vi "Untitled 8.vi"() -> ()   [LabVIEW 2009]
uses:
  <vilib>/Utility/file.llb/Read From Spreadsheet File (DBL).vi
  <vilib>/Analysis/NI_AALBase.lvlib
panel:
  in  "butter?":bool
  in  "w":dbl
  out "x/y 2":dbl
  out "x/y":dbl
  out "output cluster 3":cluster{"locations":dbl[], "locations":dbl[]}(graph)
  out "output cluster 2":cluster{"locations":dbl[], "amplitudes":dbl[]}[](graph)
  in  "threshold":dbl
  in  "offset":dbl
  in  "method":i32(ring)=1 items=["median", "noise center", "Minimum"]
  in  "number of rows (all:-1)":i32=300
  out "all rows":dbl[][](graph)
  in  "file path (dialog if empty)":path
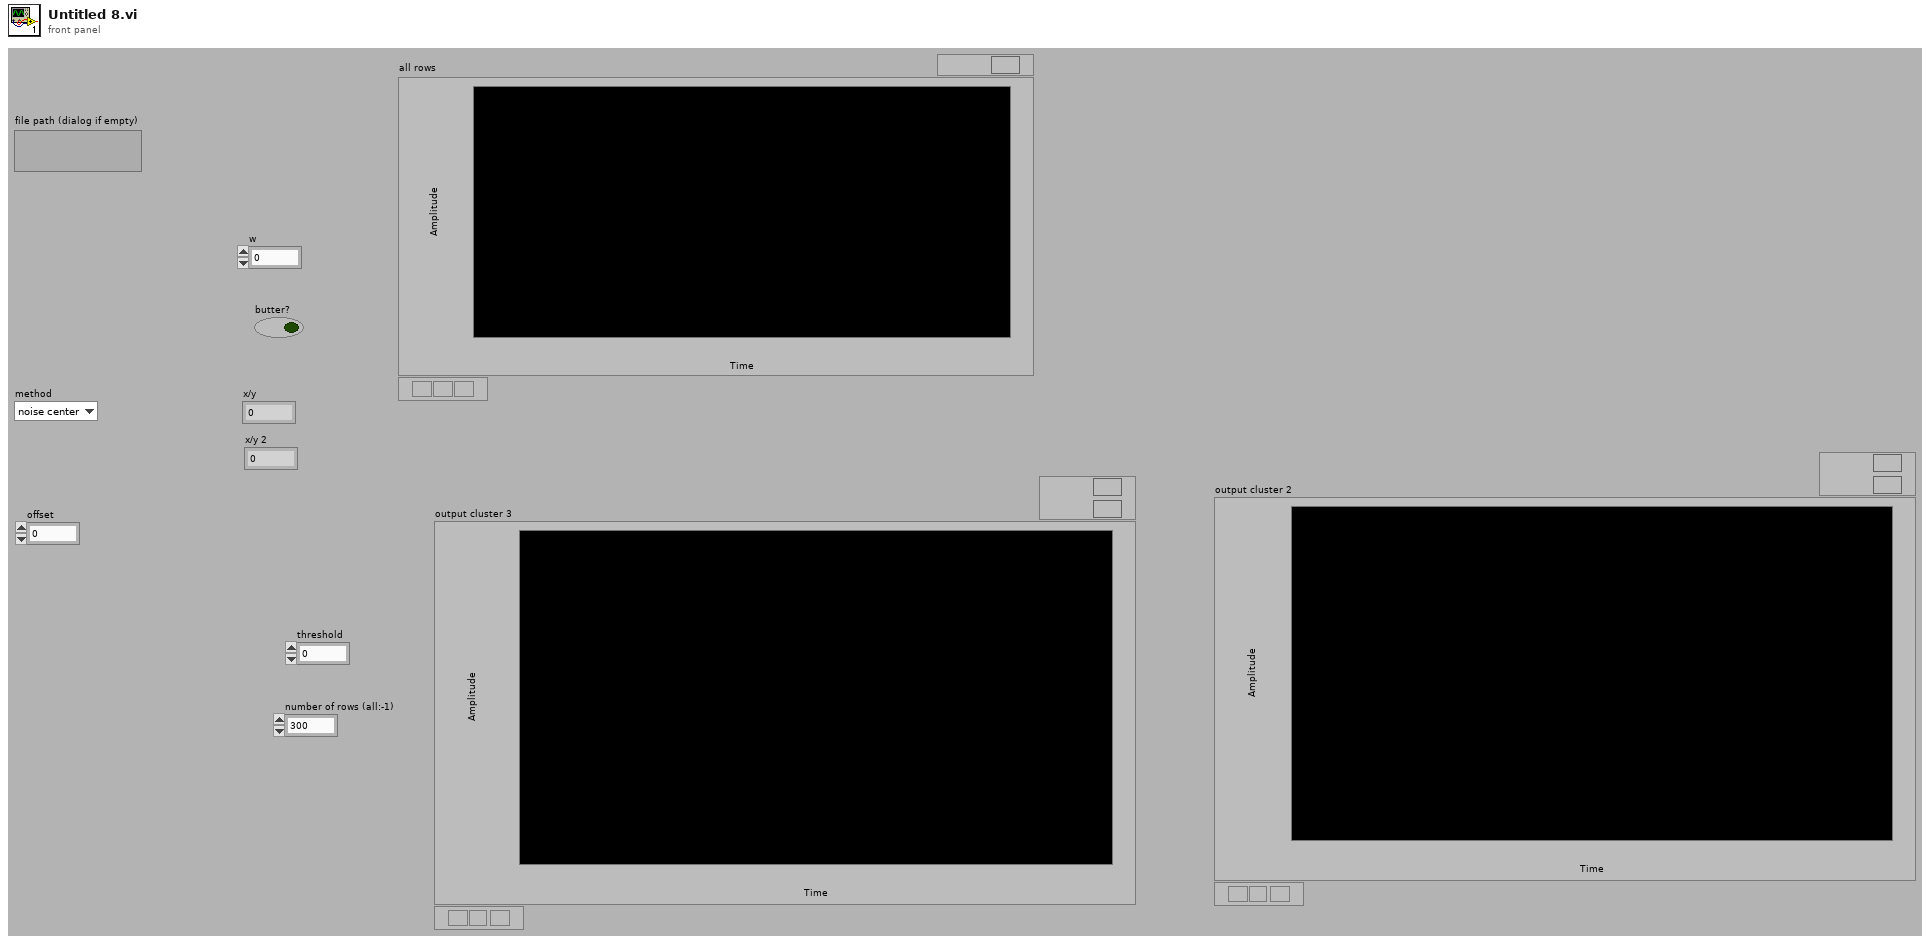
[diagram p1: front panel]
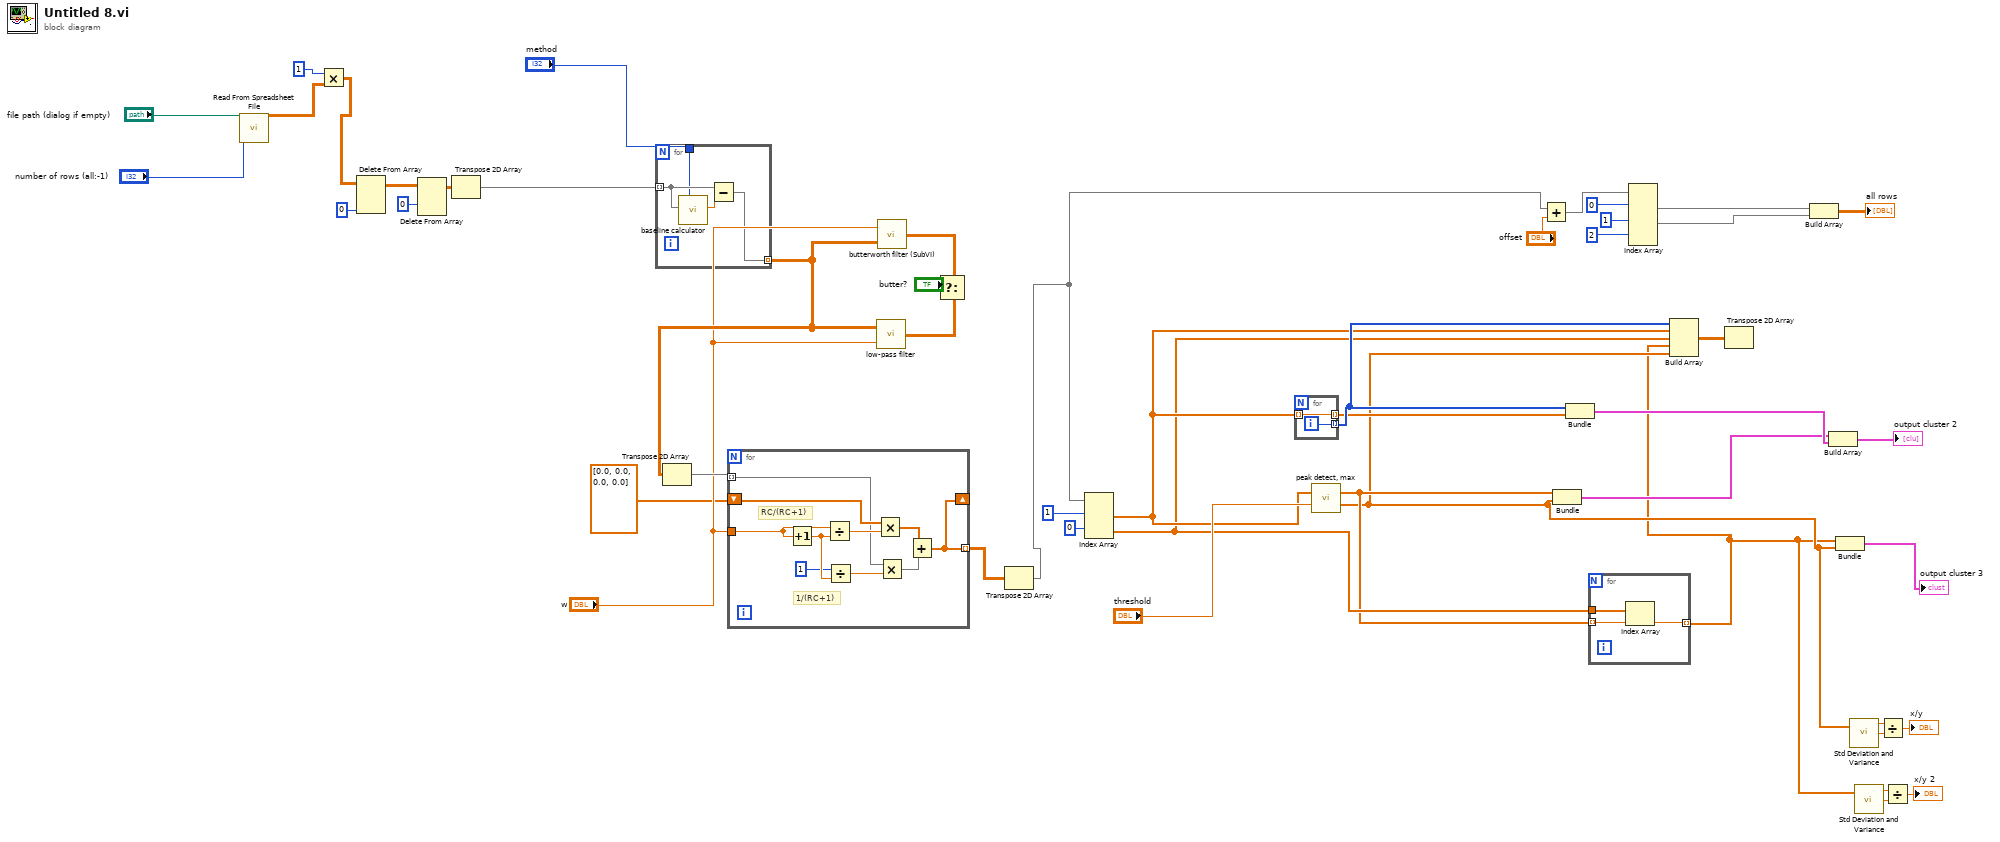
[diagram p0: block diagram]
diagram:
  n1 = call-poly <vilib>:"Read From Spreadsheet File.vi"("number of rows (all:-1)"="number of rows (all:-1)", "file path (dialog if empty)"="file path (dialog if empty)") -> ("all rows"=w35:dbl[][])  [unwired: 5 in, 4 out]
  n2 = Multiply(x=1 ("disabled index (col)"), y=w35) -> (x*y=w34:dbl[][])
  n3 = Delete From Array(array=w34, index (col)=0 ("disabled index (col)")) -> (array with subset deleted=w45:dbl[][])  [unwired: 2 in, 1 out]
  n4 = Delete From Array(array=w45, index (row)=0 ("disabled index (col)")) -> (array with subset deleted=w44:dbl[][])  [unwired: 2 in, 1 out]
  n5 = Transpose 2D Array(2D array=w44) -> (transposed array=w42:dbl[][])
  n6 = for {
    tunnel: w42 -> [w53] mode=indexing
    tunnel: "method" -> [w52]
    tunnel: [w50] -> w6 mode=indexing
    n7 = call "baseline calculator.vi"("method"=w52, "timetrace"=w53) -> ("baseline"=w51:dbl)  [unwired: 9 in]
    n8 = Subtract(x=w53, y=w51) -> (x-y=w50:dbl[])
  }
  n9 = Transpose 2D Array(2D array=w6) -> (transposed array=w5:dbl[][])
  n10 = for {
    tunnel: w5 -> [w54] mode=indexing
    tunnel: "w" -> [w57]
    tunnel: [w56] -> w2 mode=indexing
    shift-right: [w56] -> _
    shift-left: dbl[] [0.0, 0.0, 0.0, 0.0] -> [w55]
    # "1/(RC+1)"
    # "RC/(RC+1)"
    n11 = Increment(x=w57) -> (x+1=w62:dbl)
    n12 = Divide(x=w57, y=w62) -> (x/y=w61:dbl)
    n13 = Divide(x=1 ("smooth size"), y=w62) -> (x/y=w63:dbl)
    n14 = Multiply(x=w55, y=w61) -> (x*y=w59:dbl[])
    n15 = Multiply(x=w54, y=w63) -> (x*y=w60:dbl[])
    n16 = Add(x=w59, y=w60) -> (x+y=w56:dbl[])
  }
  n17 = call "low-pass filter.vi"("smooth size"="w", "Array 2"=w6) -> ("Array"=w7:dbl[][])
  n18 = call "butterworth filter (SubVI).vi"("Array 2"=w6, "w"="w") -> ("Array"=w8:dbl[][])
  n19 = Select(t=w8, s="butter?", f=w7) -> ()  [unwired: 1 out]
  n20 = Transpose 2D Array(2D array=w2) -> (transposed array=w1:dbl[][])
  n21 = Index Array(array=w1, index (row) #1=1 ("disabled index (col)"), index (row) #2=0 ("disabled index (col)")) -> (element #1=w21:dbl[], element #2=w20:dbl[])  [unwired: 2 in]
  n22 = for {
    tunnel: w21 -> [w65] mode=indexing
    tunnel: [w65] -> w22 mode=indexing
    tunnel: [w64] -> w23 mode=indexing
    i -> [w64]
  }
  n23 = call "peak detect, max.vi"("timetrace"=w21, "threshold"="threshold") -> ("locations"=w19:dbl[], "amplitudes"=w17:dbl[])  [unwired: 12 in]
  n24 = Add(x=w1, y="offset") -> (x+y=w38:dbl[][])
  n25 = Bundle("locations"=w19, "amplitudes"=w17) -> (w25:cluster{"locations":dbl[], "amplitudes":dbl[]})  [unwired: 1 in]
  n26 = Bundle(w23, w22) -> (w26:cluster{i32[], dbl[]})  [unwired: 1 in]
  n27 = for {
    tunnel: w19 -> [w68] mode=indexing
    tunnel: w20 -> [w67]
    tunnel: [w66] -> w10 mode=indexing
    n28 = Index Array(array=w67, index=w68) -> (element=w66:dbl)
  }
  n29 = Index Array(array=w38, index (row) #1=0 ("disabled index (col)"), index (row) #2=1 ("disabled index (col)"), index (row) #3=2 ("disabled index (col)")) -> (element #1=w33:dbl[], element #2=w32:dbl[])  [unwired: 3 in, 1 out]
  n30 = Build Array(w23, w21, w20, w10, w17) -> (w18:dbl[][])
  n31 = Transpose 2D Array(2D array=w18) -> ()  [unwired: 1 out]
  n32 = Build Array(w33, w32) -> (→"all rows":dbl[][])
  n33 = Build Array(w25, w26) -> (→"output cluster 2":cluster{"locations":dbl[], "amplitudes":dbl[]}[])
  n34 = Bundle(w10, "amplitudes"=w17) -> (→"output cluster 3":cluster{dbl[], "amplitudes":dbl[]})  [unwired: 1 in]
  n35 = call <vilib>:"Std Deviation and Variance.vi"("X"=w17) -> ("mean"=w16:dbl, "standard deviation"=w15:dbl)  [unwired: 1 in, 1 out]
  n36 = call <vilib>:"Std Deviation and Variance.vi"("X"=w10) -> ("mean"=w11:dbl, "standard deviation"=w12:dbl)  [unwired: 1 in, 1 out]
  n37 = Divide(x=w16, y=w15) -> (x/y=→"x/y":dbl)
  n38 = Divide(x=w11, y=w12) -> (x/y=→"x/y 2":dbl)
